vi "Tag String.vi"(4 "String In":string, 6 "String name":string) -> (0 "Stop":string, 1 "Start":string, 2 "Start Tagged String Out":string)   [LabVIEW 2014]
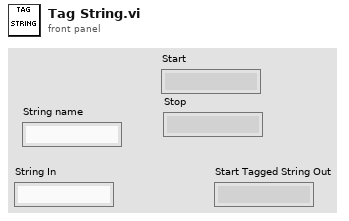
[diagram p1: front panel]
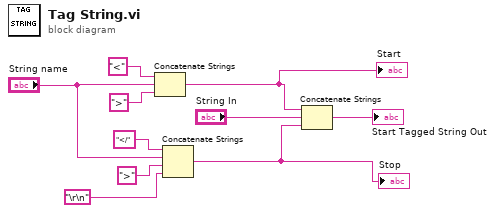
[diagram p0: block diagram]
diagram:
  n1 = Concatenate Strings("<" ("string"), "String name", ">" ("string")) -> (w3:string)
  "Start" <- w3
  n2 = Concatenate Strings("</" ("string"), "String name", ">" ("string"), "\r\n") -> (w2:string)
  "Stop" <- w2
  n3 = Concatenate Strings(w3, "String In", w2) -> (→"Start Tagged String Out":string)
